vi "mean.vi"(5 "temperatura":dbl, 7 "Array in":dbl[](array[numeric])) -> (0 "min value":dbl, 1 "max value":dbl, 2 "Array out":dbl[](array[numeric]), 3 "average":dbl)   [LabVIEW 2021]
panel:
  out "output array":dbl[](array[numeric])
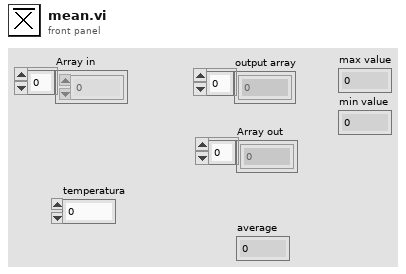
[diagram p1: front panel]
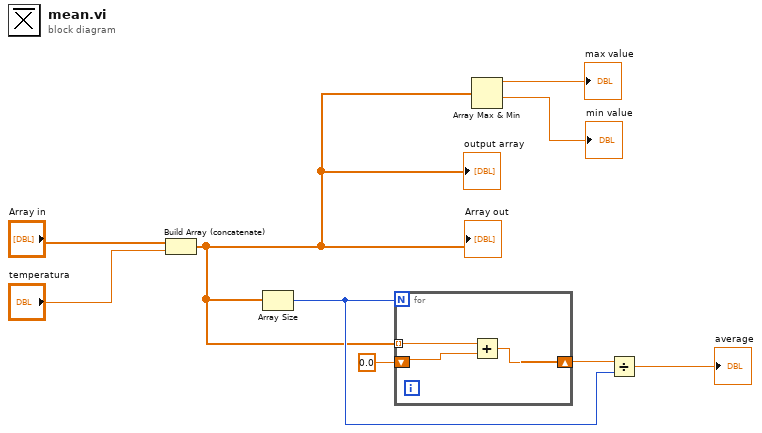
[diagram p0: block diagram]
diagram:
  n1 = Build Array (concatenate)("Array in", "temperatura") -> (w1:dbl[])
  "Array out" <- w1
  "output array" <- w1
  n2 = Array Size(array=w1) -> (size(s)=w8:i32)
  n3 = for {
    N: w8 -> [_]
    tunnel: w1 -> [w12] mode=indexing
    shift-right: [w10] -> w7
    shift-left: 0.0 -> [w11]
    n4 = Add(x=w12, y=w11) -> (x+y=w10:dbl)
  }
  n5 = Array Max & Min(array=w1) -> (max value=→"max value":dbl, min value=→"min value":dbl)  [unwired: 2 out]
  n6 = Divide(x=w7, y=w8) -> (x/y=→"average":dbl)
